vi "Recursive Find LVClasses.vi"(8 "error in (no error)":errorcluster, 11 "reference":refnum<vi>) -> (0 "error out":errorcluster, 3 "Class References":refnum<vi>[](array[refnum]))   [LabVIEW 2020, in "LUnit Test Suite.lvclass"]
uses:
  LUnit Test Suite.lvclass
  LUnit Test Suite.lvclass/LUnit Test Suite.ctl
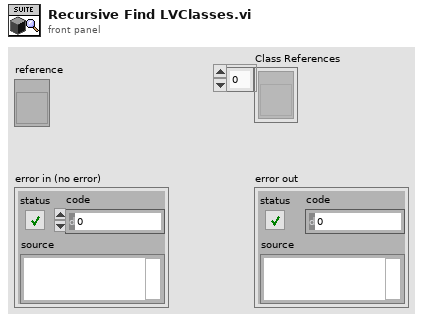
[diagram p1: front panel]
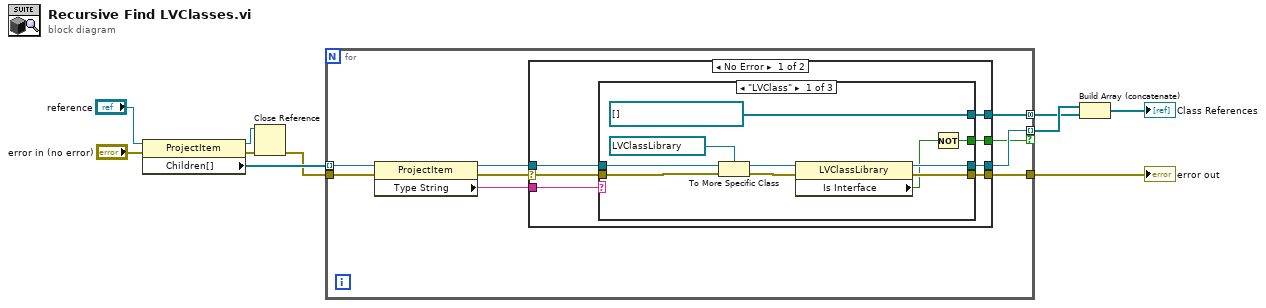
[diagram p0: block diagram]
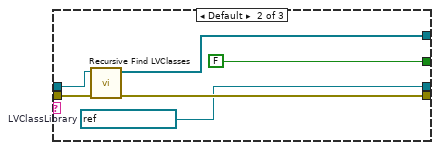
[diagram p2: hidden frame]
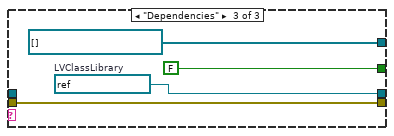
[diagram p3: hidden frame]
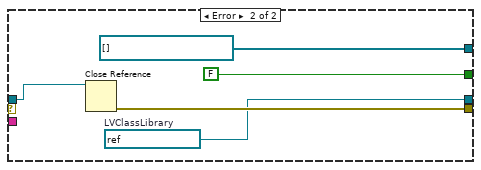
[diagram p4: hidden frame]
diagram:
  n1 = property class="ProjectItem"(reference="reference", error in="error in (no error)") -> (reference out=w1:refnum<vi>, error out=w8:errorcluster, "Children[]"=w6:refnum<vi>[])
  n2 = Close Reference(reference=w1, error in (no error)=w8) -> (error out=w2:errorcluster)
  n3 = for {
    tunnel: w6 -> [w19] mode=indexing
    tunnel: [w14] -> w9 mode=indexing if=w13
    tunnel: w2 -> [w18]
    tunnel: [w16] -> w10
    tunnel: [w12] -> w3 mode=concatenating
    n4 = property class="ProjectItem"(reference=w19, error in=w18) -> (reference out=w15:refnum<vi>, error out=w17:errorcluster, "Type String"=w11:string)
    n5 = case shown="No Error" w17 {
      selector: w17 -> [w26 _]
      tunnel: [w25 w50] -> w16
      tunnel: w15 -> [w24 w51]
      tunnel: [w23 w47] -> w14
      tunnel: w11 -> [w22 _]
      tunnel: [w21 FALSE] -> w13
      tunnel: [w20 refnum<vi>[] [] ("Class References")] -> w12
      frame No Error {
        n6 = case shown="\"LVClass\"" w22 {
          tunnel: w26 -> [w34 w42 w46]
          tunnel: [w30 w41 w46] -> w25
          tunnel: w24 -> [w36 w40 _]
          tunnel: [w31 w37 w44] -> w23
          tunnel: [w27 FALSE FALSE] -> w21
          tunnel: [refnum<vi>[] [] ("Class References") w39 refnum<vi>[] [] ("Class References")] -> w20
          frame "LVClass" {
            n7 = To More Specific Class(target class=refnum<vi> refnum ("Class References"), reference=w36, error in=w34) -> (specific class reference=w32:refnum<vi>, error out=w29:errorcluster)
            n8 = property class="LVClassLibrary"(reference=w32, error in=w29) -> (reference out=w31:refnum<vi>, error out=w30:errorcluster, "Is Interface"=w28:bool)
            n9 = Not(x=w28) -> (.not. x?=w27:bool)
          }
          frame Default {
            w37 = refnum<vi> refnum  # LVClassLibrary
            n10 = call "Recursive Find LVClasses.vi"("error in (no error)"=w42, "reference"=w40) -> ("error out"=w41:errorcluster, "Class References"=w39:refnum<vi>[])  [unwired: 8 in]
          }
          frame "Dependencies" {
            w44 = refnum<vi> refnum  # LVClassLibrary
          }
        }
      }
      frame Error {
        w47 = refnum<vi> refnum  # LVClassLibrary
        n11 = Close Reference(reference=w51) -> (error out=w50:errorcluster)  [unwired: 1 in]
      }
    }
  }
  "error out" <- w10
  n12 = Build Array (concatenate)(w9, w3) -> (→"Class References":refnum<vi>[])
